vi "Stop Core.vi"(10 "final error code":i32, 11 "Operator UI Actor in":refnum<class "Controller UI.lvclass">) -> (3 "Operator UI Actor out":refnum<class "Controller UI.lvclass">)   [LabVIEW 2016, in "Controller UI.lvlib" / "Controller UI.lvclass"]
uses:
  <userlib>/Common Components/Controller UI/Controller UI.lvclass
  <userlib>/Common Components/Controller UI/Controller UI.lvclass/Controller UI.ctl
  <userlib>/Common Components/Controller UI/Accessors/Write HW_DEV Subpanel.vi
  <userlib>/Common Components/Controller UI/Accessors/Write Subpanel VI Refnum.vi
  <userlib>/Common Components/Controller UI/Accessors/Read HW_DEV Subpanel.vi
  <userlib>/Common Components/Controller UI/Accessors/Read Subpanel VI Refnum.vi
  <userlib>/Common Components/User Interface/UI.lvclass
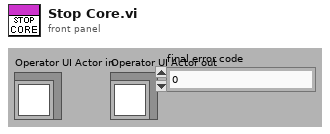
[diagram p1: front panel]
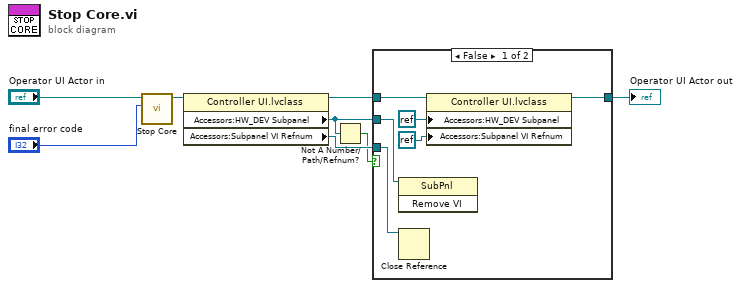
[diagram p0: block diagram]
diagram:
  n1 = call-parent "Stop Core.vi"("final error code"="final error code", "UI in"="Operator UI Actor in") -> ("UI out"=w6:refnum<class "Controller UI.lvclass">)  [unwired: 9 in]
  n2 = property class="Controller UI.lvclass"(reference=w6) -> (reference out=w5:refnum<class "Controller UI.lvclass">, "Accessors:HW_DEV Subpanel"=w2:refnum<vi>, "Accessors:Subpanel VI Refnum"=w4:refnum<vi>)  [unwired: 1 in, 1 out]
  n3 = Not A Number/Path/Refnum?(number/path/refnum=w2) -> (NaN/Path/Refnum?=w1:bool)
  n4 = case shown="False" w1 {
    tunnel: w5 -> [w14 w15]
    tunnel: w4 -> [w13 _]
    tunnel: [w12 w15] -> w3
    tunnel: w2 -> [w9 _]
    frame False {
      n5 = invoke class="SubPnl" method="Remove VI"(reference=w9) -> ()  [unwired: 2 in, 3 out]
      n6 = Close Reference(reference=w13) -> ()  [unwired: 1 in, 1 out]
      n7 = property class="Controller UI.lvclass"(reference=w14, "Accessors:HW_DEV Subpanel"=refnum<k0> refnum, "Accessors:Subpanel VI Refnum"=refnum<k0> refnum) -> (reference out=w12:refnum<class "Controller UI.lvclass">)  [unwired: 1 in, 1 out]
    }
    frame True {
    }
  }
  "Operator UI Actor out" <- w3
